vi "PointGrey Grasshopper_Settings.vi"(0 "Camera References":T4[](array[typedef]), 1 "Offset and gain":dbl[][](array[numeric]), 5 "Camera to address":i32 min=0 max=1 step=1, 7 "Camera orientation":T3(array[ring])=[enum."No rotation, No flip", enum."No rotation, No flip", enum."No rotation, Flip LR"], 9 "Which cameras record":bool[](array[boolean]), 11 "RGB Channels in":T2(array[ring]), 12 "Image buffers":T1[](array[typedef])) -> (3 "Offset gain out":dbl[][](array[numeric]), 6 "Camera to address out":i32, 8 "Camera orientation out":T3(array[ring])=[enum."No rotation, No flip", enum."No rotation, No flip", enum."No rotation, Flip LR"], 10 "Which cameras record out":bool[](array[boolean]), 15 "RGB Channels out":T2(array[ring]))   [LabVIEW 2018]
uses:
  <vilib>/userdefined/High Color/IMAQdx.ctl
  <vilib>/vision/Image Controls.llb/IMAQ Image.ctl
  <vilib>/Utility/miscctls.llb/LVOutOfRangeActionTypeDef.ctl
  <vilib>/vision/driver/IMAQdx.llb/IMAQdx Attribute Visibility.ctl
  <vilib>/vision/driver/NI_Vision_Acquisition_Software.lvlib
  <resource>/objmgr/imaqdx.rc
panel:
  in  "Tab Control":enum32{"Settings", "RGB"}(tab)
  in  "Refresh":bool
  in  "Tree":string(tree)
  in  "CameraU32":u32
  in  "CameraI64":i64
  in  "CameraDBL":dbl
  in  "CameraString":string
  in  "CameraBool":bool
  in  "CameraEnum":u16(ring) items=["Off", "Once", "Continuous"]
  in  "CameraCommand":string
  in  "Autorange Blue":bool
  in  "Autorange Green":bool
  in  "Autorange Red":bool
  in  "OK Button":bool
  # "Camera 0 is RGB, Camera 1,2... are individual cameras"
  # "Offset"
  # "Gain"
  # "Red"
  # "Green"
  # "Blue"
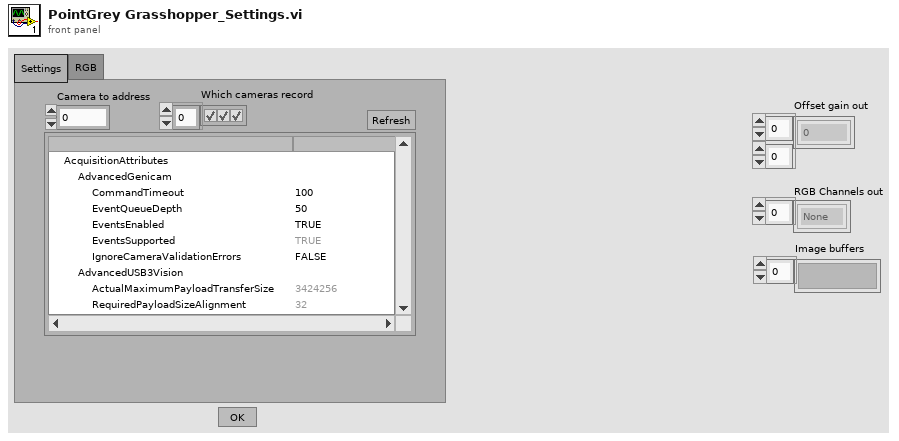
[diagram p1: front panel]
types:
  T1 = typedef "IMAQ Image.ctl" = refnum<image>
  T2 = enum16{"None", "Camera 1", "Camera 2", "Camera 3"}[]
  T3 = enum16{"No rotation, No flip", "No rotation, Flip UD", "No rotation, Flip LR", "Clockwise, No flip", "Clockwise, Flip UD", "Clockwise, Flip LR", "Anticlockwise, No flip", "Anticlockwise, Flip UD", "Anticlockwise, Flip LR"}[]
  T4 = typedef "IMAQdx.ctl" = refnum<k21>
  T5 = typedef "LVOutOfRangeActionTypeDef.ctl" = cluster{"Out of Range Action Minimum":u8, "Out of Range Action Maximum":u8, "Out of Range Action Increment":u8}
  T6 = typedef "NI_Vision_Acquisition_Software.lvlib/IMAQdx Attribute Visibility.ctl" = enum32{"Simple", "Intermediate", "Advanced"}
  T7 = enum8{"Enabled", "Disabled", "Disabled and Grayed Out"}
  T8 = typedef "NI_Vision_Acquisition_Software.lvlib/IMAQdx Attribute Type.ctl" = enum32{"U32", "I64", "DBL", "String", "Enum", "Bool", "Command"}
  T9 = cluster{"Attribute Type":T8, "Readable":bool, "Writable":bool, "Attribute Name":string}[]
  T10 = enum16{"None", "Camera 1", "Camera 2", "Camera 3"}
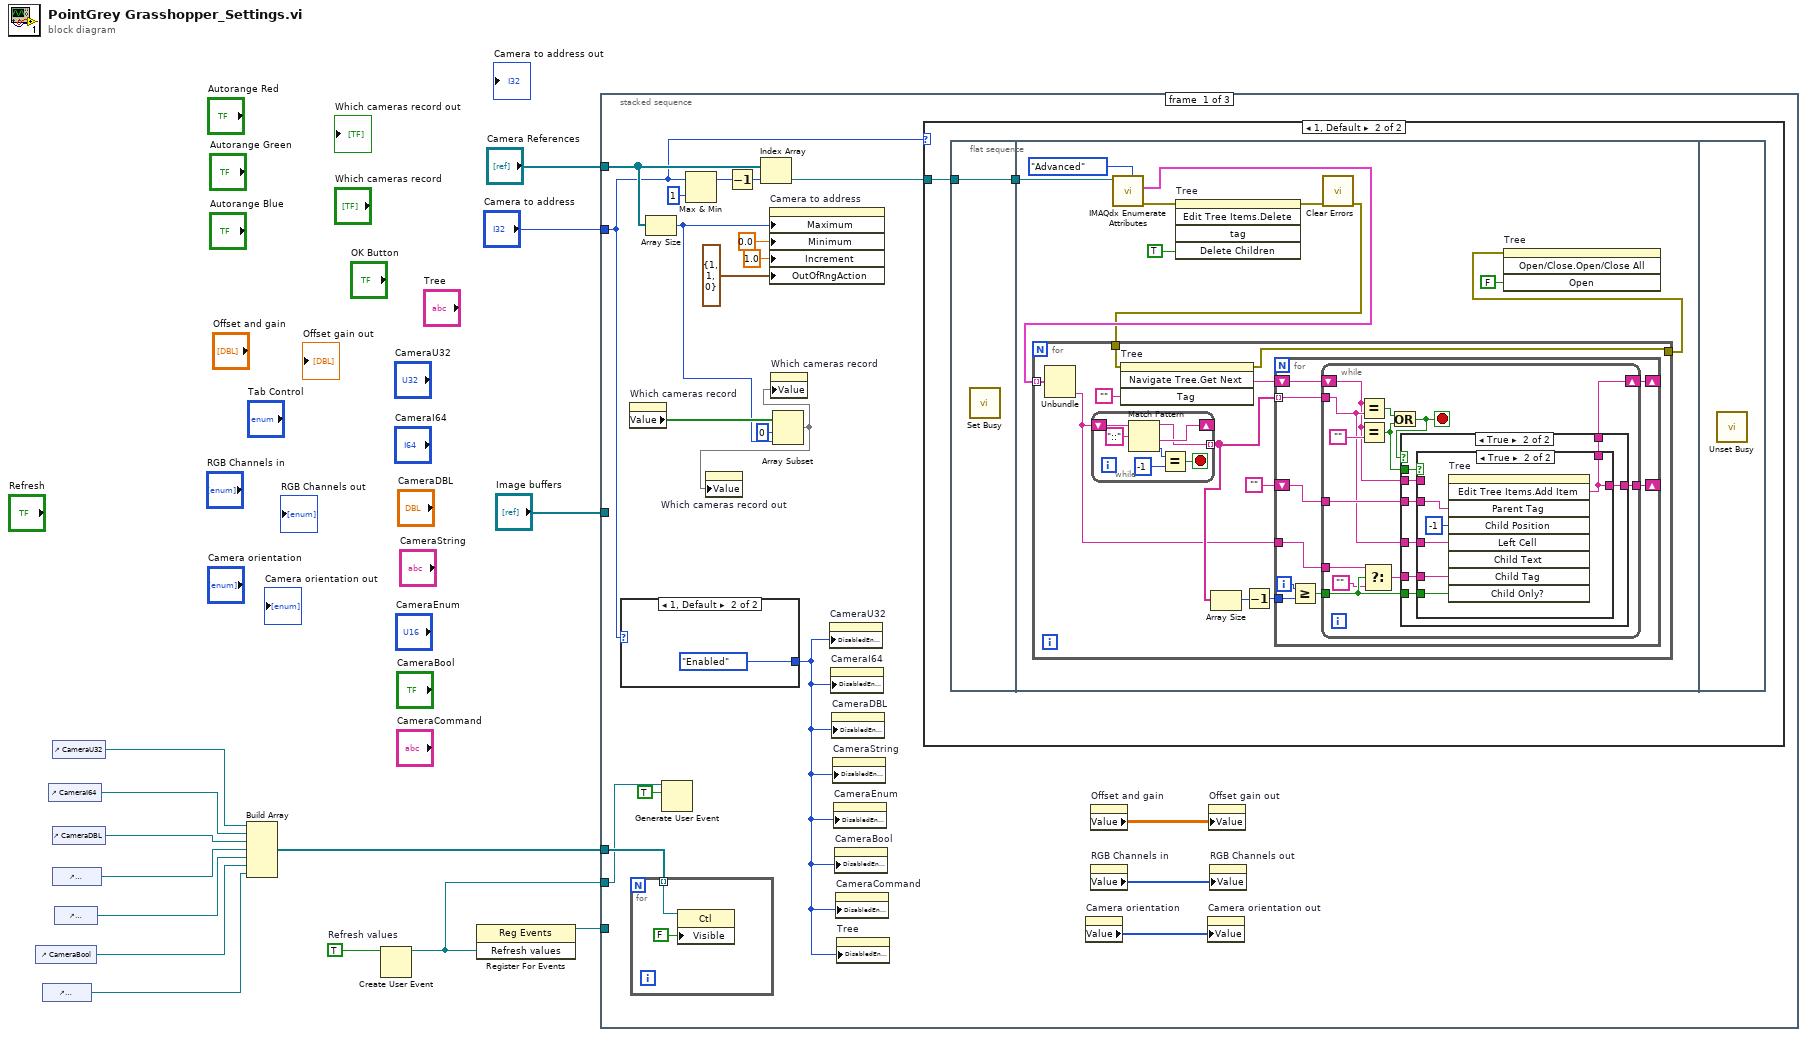
[diagram p0: block diagram]
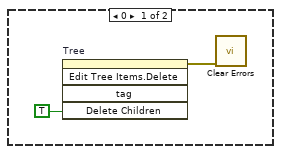
[diagram p2: hidden frame]
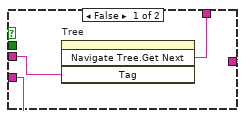
[diagram p3: hidden frame]
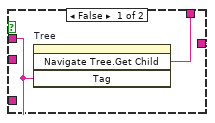
[diagram p4: hidden frame]
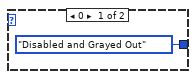
[diagram p5: hidden frame]
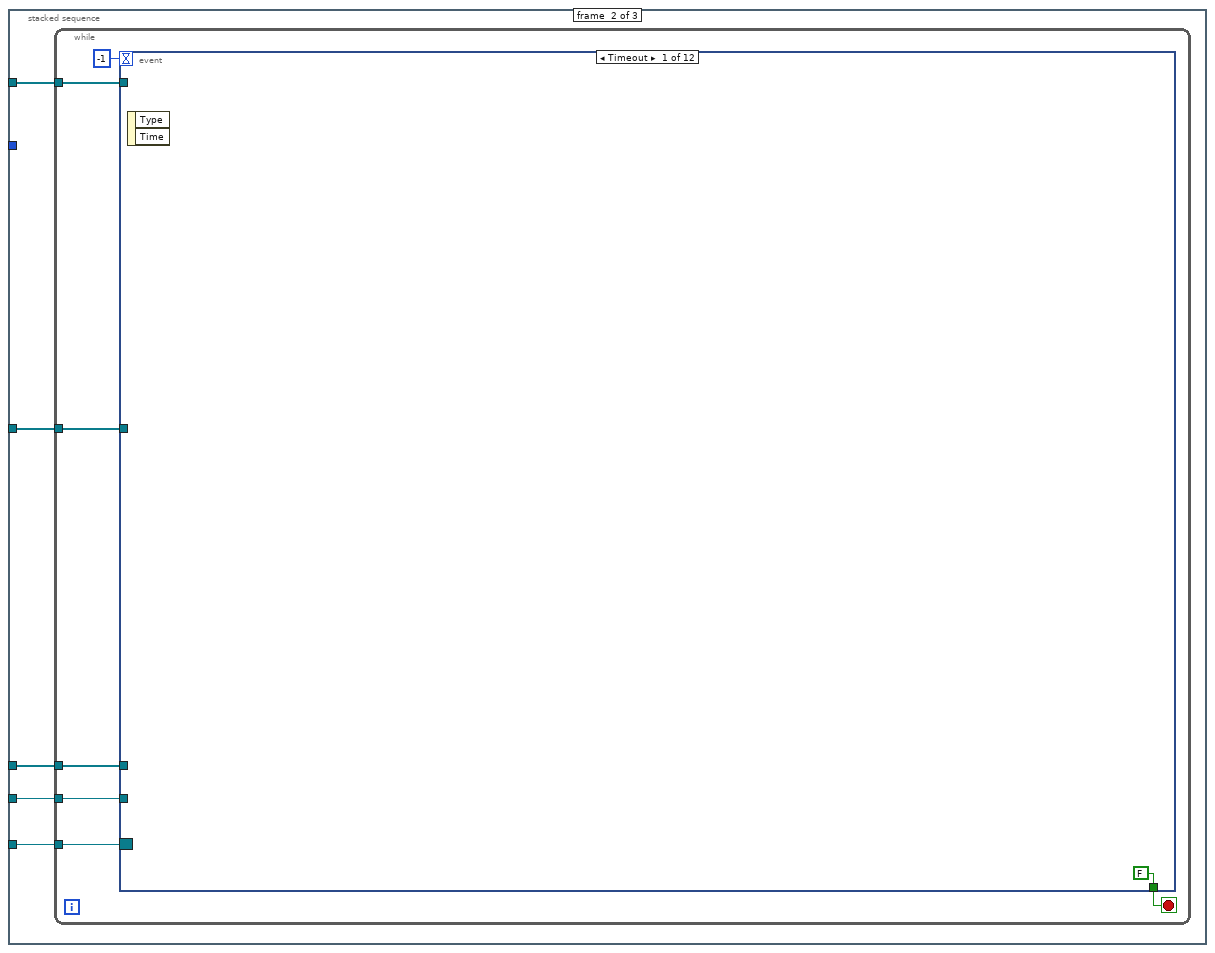
[diagram p6: hidden frame]
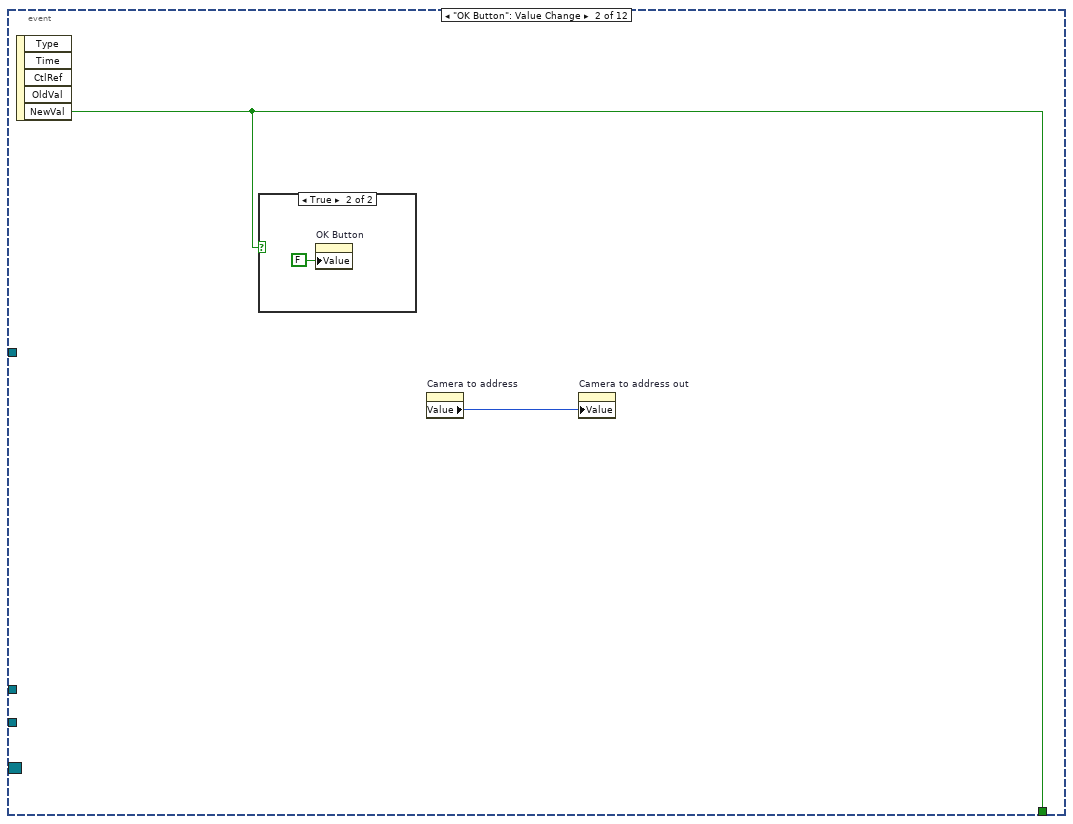
[diagram p7: hidden frame]
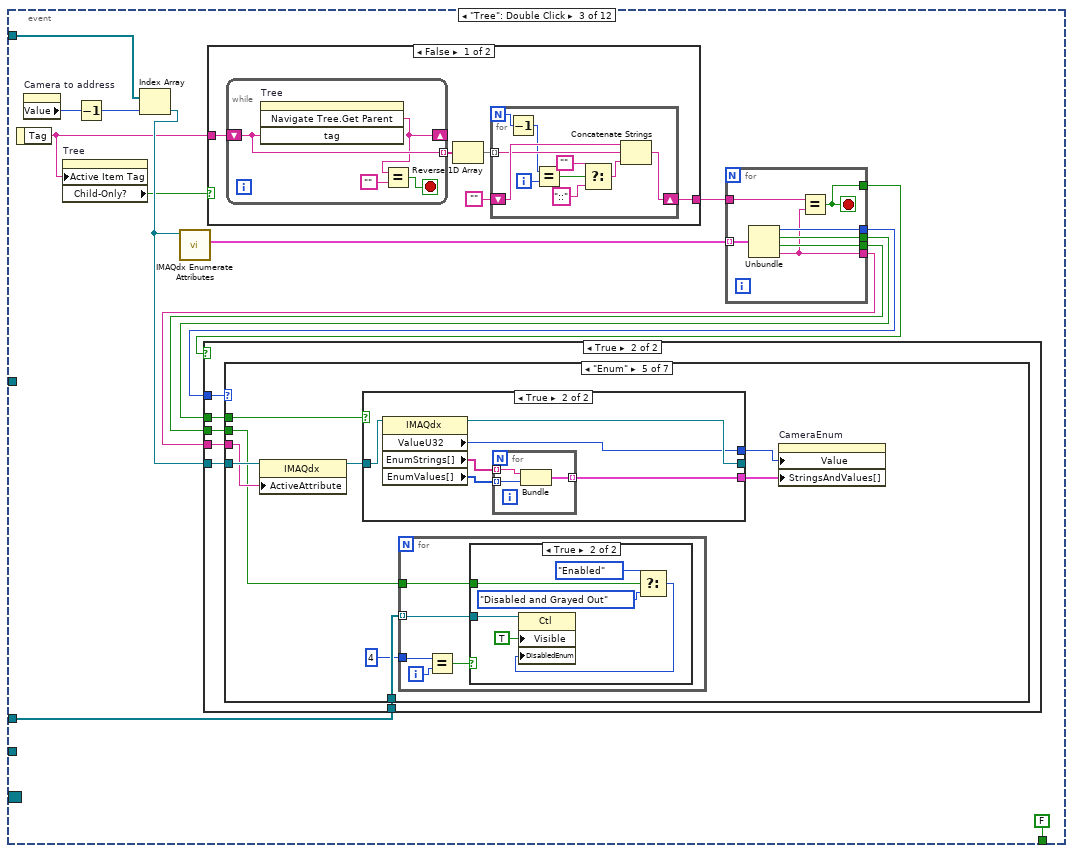
[diagram p9: hidden frame]
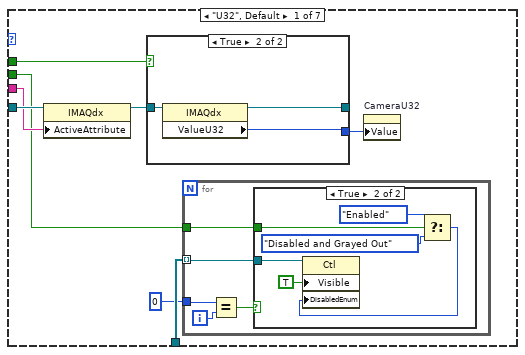
[diagram p12: hidden frame]
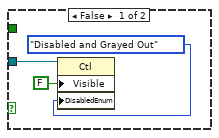
[diagram p13: hidden frame]
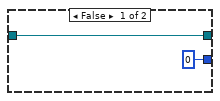
[diagram p14: hidden frame]
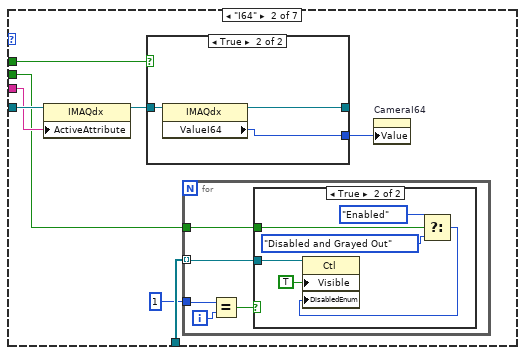
[diagram p15: hidden frame]
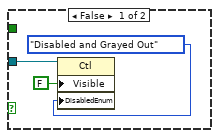
[diagram p16: hidden frame]
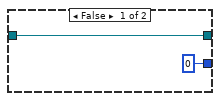
[diagram p17: hidden frame]
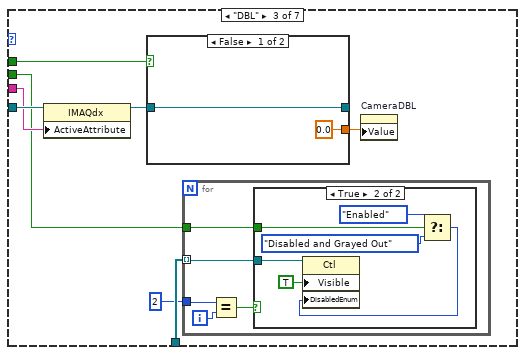
[diagram p18: hidden frame]
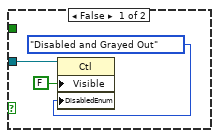
[diagram p19: hidden frame]
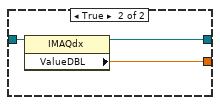
[diagram p20: hidden frame]
diagram:
  w2 = TRUE  # Refresh values
  n1 = control-ref of="CameraBool"() -> (w7:refnum<vi>)
  n2 = control-ref of="CameraCommand"() -> (w6:refnum<vi>)
  n3 = control-ref of="CameraI64"() -> (w11:refnum<vi>)
  n4 = control-ref of="CameraU32"() -> (w12:refnum<vi>)
  n5 = control-ref of="CameraDBL"() -> (w10:refnum<vi>)
  n6 = control-ref of="CameraString"() -> (w9:refnum<vi>)
  n7 = control-ref of="CameraEnum"() -> (w8:refnum<vi>)
  n8 = Build Array(w12, w11, w10, w9, w8, w7, w6) -> (w5:refnum<vi>[])
  n9 = Create User Event(user event datatype=w2) -> (user event=w1:refnum<user-event>)  [unwired: 1 in, 1 out]
  n10 = register-events(w1) -> (reference out=w3:refnum<event-registration>)  [unwired: 2 in, 1 out]
  n11 = stacked-sequence {
    tunnel: "Camera References" -> [w32 w115 _]
    tunnel: "Camera to address" -> [w15 _ _]
    tunnel: w5 -> [w33 w114 _]
    tunnel: "Image buffers" -> [_ w113 _]
    tunnel: w3 -> [_ w112 _]
    tunnel: w1 -> [w21 w111 w650]
    frame #0 {
      n12 = case shown="1, Default" w15 {
        tunnel: [T7."Disabled and Grayed Out" ("Disabled") T7."Enabled" ("Disabled")] -> w26
        frame 0 {
        }
        frame 1, Default {
        }
      }
      n13 = property on="Which cameras record" class="Arr (strict)"() -> ("Value"=w27:bool[])  [unwired: 2 in, 2 out]
      n14 = for {
        tunnel: w33 -> [w110] mode=indexing
        n15 = property class="Ctl"(reference=w110, "Visible"=FALSE) -> ()  [unwired: 1 in, 2 out]
      }
      n16 = Array Size(array=w32) -> (size(s)=w22:i32)
      n17 = Generate User Event(user event=w21, event data cluster=TRUE ("event data")) -> ()  [unwired: 2 in, 2 out]
      n18 = Max & Min(x=w15, y=1) -> (max(x,y)=w17:i32)  [unwired: 1 out]
      n19 = Decrement(x=w17) -> (x-1=w19:i32)
      n20 = Index Array(array=w32, index=w19) -> (element=w34:T4)
      n21 = property on="Camera to address" class="DigNum (strict)"("Maximum"=w22, "Minimum"=0.0 ("Data Entry Limits:Minimum"), "Increment"=1.0 ("Data Entry Limits:Increment"), "OutOfRngAction"=T5 {"Out of Range Action Minimum"=1, "Out of Range Action Maximum"=1, "Out of Range Action Increment"=0} ("Response to Value Outside Limits")) -> ()  [unwired: 2 in, 2 out]
      n22 = Array Subset(array=w27, index=0, length=w22) -> (w18:bool[])
      n23 = property on="Which cameras record out" class="Arr (strict)"("Value"=w18) -> ()  [unwired: 2 in, 2 out]
      n24 = property on="Which cameras record" class="Arr (strict)"("Value"=w18) -> ()  [unwired: 2 in, 2 out]
      n25 = property on="CameraU32" class="DigNum (strict)"("DisabledEnum"=w26) -> ()  [unwired: 2 in, 2 out]
      n26 = property on="CameraI64" class="DigNum (strict)"("DisabledEnum"=w26) -> ()  [unwired: 2 in, 2 out]
      n27 = property on="CameraDBL" class="DigNum (strict)"("DisabledEnum"=w26) -> ()  [unwired: 2 in, 2 out]
      n28 = property on="CameraString" class="Str"("DisabledEnum"=w26) -> ()  [unwired: 2 in, 2 out]
      n29 = property on="CameraEnum" class="Ring (strict)"("DisabledEnum"=w26) -> ()  [unwired: 2 in, 2 out]
      n30 = property on="CameraBool" class="Bool (strict)"("DisabledEnum"=w26) -> ()  [unwired: 2 in, 2 out]
      n31 = property on="CameraCommand" class="Str"("DisabledEnum"=w26) -> ()  [unwired: 2 in, 2 out]
      n32 = property on="Tree" class="Tree (strict)"("DisabledEnum"=w26) -> ()  [unwired: 2 in, 2 out]
      n33 = case shown="1, Default" w15 {
        tunnel: w34 -> [_ w38]
        frame 0 {
          n34 = invoke on="Tree" class="Tree (strict)" method="Edit Tree Items.Delete"("Delete Children"=TRUE ("Delete Children?")) -> (error out=w35:errorcluster)  [unwired: 4 in, 4 out]
          n35 = call <vilib>:"Clear Errors.vi"("error in (no error)"=w35) -> ()  [unwired: 5 in, 2 out]
        }
        frame 1, Default {
          n36 = flat-sequence {
            tunnel: w38 -> [w39]
            tunnel: [w39] -> w37
            tunnel: w37 -> [w40]
            frame #0 {
              n37 = call <vilib>:"Set Busy.vi"() -> ()  [unwired: 10 in, 2 out]
            }
            frame #1 {
              n38 = call <vilib>:"IMAQdx Enumerate Attributes.vi"("Visibility"=IMAQdx_Attribute_Visibility."Advanced", "Session In"=w40) -> ("error out"=w44:errorcluster, "Attribute Information Array"=w48:T9)  [unwired: 7 in, 1 out]
              n39 = invoke on="Tree" class="Tree (strict)" method="Edit Tree Items.Delete"(error in=w44, "Delete Children"=TRUE ("Delete Children?")) -> (error out=w43:errorcluster)  [unwired: 3 in, 4 out]
              n40 = call <vilib>:"Clear Errors.vi"("error in (no error)"=w43) -> ("error out"=w45:errorcluster)  [unwired: 5 in, 1 out]
              n41 = for {
                tunnel: w48 -> [w58] mode=indexing
                tunnel: w45 -> [w51]
                tunnel: [w50] -> w47
                n42 = Unbundle(w58) -> ("Attribute Name"=w49:string)  [unwired: 3 out]
                n43 = while {
                  shift-right: [w104] -> _
                  shift-left: w49 -> [w106]
                  tunnel: [w100] -> w55 mode=indexing
                  stop <- w101 stop-if-true
                  n44 = Match Pattern(string=w106, regular expression="::") -> (before substring=w100:string, after substring=w104:string, offset past match=w103:i32)  [unwired: 1 in, 1 out]
                  n45 = Equal?(x=w103, y=-1) -> (x = y?=w101:bool)
                }
                n46 = invoke on="Tree" class="Tree (strict)" method="Navigate Tree.Get Next"(error in=w51, "Tag"="") -> (error out=w50:errorcluster, "Navigate Tree:Get Next Item"=w53:string)  [unwired: 2 in, 2 out]
                n47 = Array Size(array=w55) -> (size(s)=w56:i32)
                n48 = Decrement(x=w56) -> (x-1=w52:i32)
                n49 = for {
                  tunnel: w55 -> [w67] mode=indexing
                  shift-right: [w66] -> _
                  shift-left: "" -> [w65]
                  tunnel: w52 -> [w63]
                  shift-right: [w60] -> _
                  shift-left: w53 -> [w61]
                  tunnel: w49 -> [w59]
                  i -> [w62]
                  n50 = Greater Or Equal?(x=w62, y=w63) -> (x >= y?=w64:bool)
                  n51 = while {
                    shift-right: [w72] -> w60
                    shift-left: w61 -> [w73]
                    tunnel: w67 -> [w74]
                    tunnel: [w76] -> w66
                    tunnel: w65 -> [w75]
                    tunnel: w64 -> [w71]
                    tunnel: w59 -> [w69]
                    stop <- w78 stop-if-true
                    n52 = Equal?(x=w73, y=w74) -> (x = y?=w79:bool)
                    n53 = Equal?(x=w73, y="") -> (x = y?=w77:bool)
                    n54 = Select(t=w69, s=w71, f="") -> (s? t:f=w70:string)
                    n55 = Or(x=w79, y=w77) -> (x .or. y?=w78:bool)
                    n56 = case shown="True" w78 {
                      tunnel: w73 -> [w82 w90]
                      tunnel: w77 -> [_ w91]
                      tunnel: [w83 w89] -> w76
                      tunnel: w75 -> [w83 w88]
                      tunnel: w71 -> [_ w87]
                      tunnel: w74 -> [_ w86]
                      tunnel: [w81 w85] -> w72
                      tunnel: w70 -> [_ w84]
                      frame False {
                        n57 = invoke on="Tree" class="Tree (strict)" method="Navigate Tree.Get Next"("Tag"=w82) -> ("Navigate Tree:Get Next Item"=w81:string)  [unwired: 3 in, 3 out]
                      }
                      frame True {
                        n58 = case shown="True" w91 {
                          tunnel: w90 -> [w92 _]
                          tunnel: [w92 w95] -> w89
                          tunnel: w88 -> [_ w96]
                          tunnel: w87 -> [_ w98]
                          tunnel: w86 -> [_ w97]
                          tunnel: [w93 w95] -> w85
                          tunnel: w84 -> [_ w94]
                          frame False {
                            n59 = invoke on="Tree" class="Tree (strict)" method="Navigate Tree.Get Child"("Tag"=w92) -> ("Navigate Tree:Get Child"=w93:string)  [unwired: 3 in, 3 out]
                          }
                          frame True {
                            n60 = invoke on="Tree" class="Tree (strict)" method="Edit Tree Items.Add Item"("Parent Tag"=w96, "Child Position"=-1, "Left Cell"=w97, "Child Tag"=w94, "Child Only?"=w98) -> ("Edit Tree Items:Add Item"=w95:string)  [unwired: 4 in, 8 out]
                          }
                        }
                      }
                    }
                  }
                }
              }
              n61 = invoke on="Tree" class="Tree (strict)" method="Open/Close.Open/Close All"(error in=w47, "Open"=FALSE ("Open?")) -> ()  [unwired: 2 in, 4 out]
            }
            frame #2 {
              n62 = call <vilib>:"Unset Busy.vi"() -> ()  [unwired: 11 in, 1 out]
            }
          }
        }
      }
      n63 = property on="Camera orientation" class="Arr (strict)"() -> ("Value"=w16:T3)  [unwired: 2 in, 2 out]
      n64 = property on="Offset and gain" class="Arr (strict)"() -> ("Value"=w24:dbl[][])  [unwired: 2 in, 2 out]
      n65 = property on="RGB Channels in" class="Arr (strict)"() -> ("Value"=w23:T2)  [unwired: 2 in, 2 out]
      n66 = property on="Camera orientation out" class="Arr (strict)"("Value"=w16) -> ()  [unwired: 2 in, 2 out]
      n67 = property on="Offset gain out" class="Arr (strict)"("Value"=w24) -> ()  [unwired: 2 in, 2 out]
      n68 = property on="RGB Channels out" class="Arr (strict)"("Value"=w23) -> ()  [unwired: 2 in, 2 out]
    }
    frame #1 {
      n69 = while {
        tunnel: w115 -> [w120]
        tunnel: w114 -> [w119]
        tunnel: w113 -> [w118]
        tunnel: w112 -> [w117]
        tunnel: w111 -> [w116]
        stop <- w121 stop-if-true
        n70 = event shown="[0] Timeout" {
          selector: w117 -> [_ _ _ _ _ _ _ _ _ _ _ _]
          dyn-events: _ -> [_ _ _ _ _ _ _ _ _ _ _ _]
          timeout: -1 -> [_ _ _ _ _ _ _ _ _ _ _ _]
          tunnel: [FALSE ("NewVal") w125 FALSE ("NewVal") FALSE ("NewVal") FALSE ("NewVal") FALSE ("NewVal") FALSE ("NewVal") FALSE ("NewVal") FALSE ("NewVal") FALSE ("NewVal") FALSE ("NewVal") FALSE ("NewVal")] -> w121
          tunnel: w120 -> [_ _ w134 w373 w458 w464 _ _ _ _ w598 _]
          tunnel: w119 -> [_ _ w131 _ _ _ _ _ _ _ w600 _]
          tunnel: w118 -> [_ _ _ _ _ _ _ _ _ w553 _ _]
          tunnel: w116 -> [_ _ _ _ _ w460 _ _ _ _ w596 w645]
          event Timeout {
            n71 = event-data() -> ()  [unwired: 1 in, 2 out]
          }
          event "OK Button": Value Change {
            n72 = event-data() -> ("NewVal"=w125:bool)  [unwired: 1 in, 4 out]
            n73 = case shown="True" w125 {
              frame False {
              }
              frame True {
                n74 = property on="OK Button" class="Bool (strict)"("Value"=FALSE ("OK Button")) -> ()  [unwired: 2 in, 2 out]
              }
            }
            n75 = property on="Camera to address" class="DigNum (strict)"() -> ("Value"=w124:i32)  [unwired: 2 in, 2 out]
            n76 = property on="Camera to address out" class="DigNum (strict)"("Value"=w124) -> ()  [unwired: 2 in, 2 out]
          }
          event "Tree": Double Click {
            n77 = event-data() -> ("Tag"=w128:string)  [unwired: 1 in]
            n78 = property on="Camera to address" class="DigNum (strict)"() -> ("Value"=w133:i32)  [unwired: 2 in, 2 out]
            n79 = property on="Tree" class="Tree (strict)"("Active Item Tag"=w128) -> ("Child-Only?"=w127:bool)  [unwired: 2 in, 2 out]
            n80 = Decrement(x=w133) -> (x-1=w129:i32)
            n81 = Index Array(array=w134, index=w129) -> (element=w132:T4)
            n82 = call <vilib>:"IMAQdx Enumerate Attributes.vi"("Session In"=w132) -> ("Attribute Information Array"=w135:T9)  [unwired: 8 in, 2 out]
            n83 = case shown="False" w127 {
              tunnel: [w143 w161] -> w141
              tunnel: w128 -> [w142 w161]
              frame False {
                n84 = while {
                  shift-right: [w149] -> _
                  shift-left: w142 -> [w150]
                  tunnel: [w150] -> w146 mode=indexing
                  stop <- w147 stop-if-true
                  n85 = invoke on="Tree" class="Tree (strict)" method="Navigate Tree.Get Parent"("tag"=w150) -> ("Navigate Tree:Get Parent"=w149:string)  [unwired: 3 in, 3 out]
                  n86 = Equal?(x=w149, y="") -> (x = y?=w147:bool)
                }
                n87 = Reverse 1D Array(array=w146) -> (reversed array=w144:string[])
                n88 = for {
                  N -> [w157]
                  tunnel: w144 -> [w159] mode=indexing
                  shift-right: [w151] -> w143
                  shift-left: "" -> [w160]
                  i -> [w154]
                  n89 = Decrement(x=w157) -> (x-1=w155:i32)
                  n90 = Equal?(x=w155, y=w154) -> (x = y?=w156:bool)
                  n91 = Select(t="", s=w156, f="::" ("t")) -> (s? t:f=w158:string)
                  n92 = Concatenate Strings(w160, w159, w158) -> (w151:string)
                }
              }
              frame True {
              }
            }
            n93 = for {
              tunnel: w135 -> [w371] mode=indexing
              tunnel: w141 -> [w370]
              tunnel: [w369] -> w137
              tunnel: [w368] -> w138
              tunnel: [w367] -> w139
              tunnel: [w366] -> w140
              tunnel: [w365] -> w136
              stop <- w366 stop-if-true
              n94 = Unbundle(w371) -> ("Attribute Type"=w367:T8, "Readable"=w368:bool, "Writable"=w369:bool, "Attribute Name"=w365:string)
              n95 = Equal?(x=w370, y=w365) -> (x = y?=w366:bool)
            }
            n96 = case shown="True" w140 {
              tunnel: w139 -> [_ w167]
              tunnel: w138 -> [_ w166]
              tunnel: w137 -> [_ w165]
              tunnel: w136 -> [_ w164]
              tunnel: w132 -> [_ w163]
              tunnel: w131 -> [_ w162]
              frame False {
              }
              frame True {
                n97 = case shown="\"Enum\"" w167 {
                  tunnel: w166 -> [w169 w196 w223 w250 w277 w312 w339]
                  tunnel: w165 -> [w168 w195 w222 w249 w276 w311 w338]
                  tunnel: w164 -> [w174 w201 w228 w255 w283 w317 w344]
                  tunnel: w163 -> [w175 w202 w229 w256 w284 w318 w345]
                  tunnel: w162 -> [w172 w199 w226 w253 w281 w315 w342]
                  frame "U32", Default {
                    n98 = property class="IMAQdx"(reference=w175, "ActiveAttribute"=w174) -> (reference out=w173:T4)  [unwired: 1 in, 1 out]
                    n99 = case shown="True" w169 {
                      tunnel: w173 -> [w191 w194]
                      tunnel: [w191 w193] -> _
                      tunnel: [u32 0 ("ValueU32") w192] -> w170
                      frame False {
                      }
                      frame True {
                        n100 = property class="IMAQdx"(reference=w194) -> (reference out=w193:T4, "ValueU32"=w192:u32)  [unwired: 1 in, 1 out]
                      }
                    }
                    n101 = for {
                      tunnel: w172 -> [w180] mode=indexing
                      tunnel: 0 -> [w177]
                      tunnel: w168 -> [w176]
                      i -> [w179]
                      n102 = Equal?(x=w177, y=w179) -> (x = y?=w178:bool)
                      n103 = case shown="True" w178 {
                        tunnel: w180 -> [w183 w189]
                        tunnel: w176 -> [_ w187]
                        frame False {
                          n104 = property class="Ctl"(reference=w183, "Visible"=FALSE, "DisabledEnum"=T7."Disabled and Grayed Out" ("Disabled")) -> ()  [unwired: 1 in, 2 out]
                        }
                        frame True {
                          n105 = Select(t=T7."Enabled" ("Disabled"), s=w187, f=T7."Disabled and Grayed Out" ("Disabled")) -> (s? t:f=w184:T7)
                          n106 = property class="Ctl"(reference=w189, "Visible"=TRUE, "DisabledEnum"=w184) -> ()  [unwired: 1 in, 2 out]
                        }
                      }
                    }
                    n107 = property on="CameraU32" class="DigNum (strict)"("Value"=w170) -> ()  [unwired: 2 in, 2 out]
                  }
                  frame "I64" {
                    n108 = property class="IMAQdx"(reference=w202, "ActiveAttribute"=w201) -> (reference out=w200:T4)  [unwired: 1 in, 1 out]
                    n109 = case shown="True" w196 {
                      tunnel: w200 -> [w218 w221]
                      tunnel: [w218 w220] -> _
                      tunnel: [i64 0 ("ValueI64") w219] -> w197
                      frame False {
                      }
                      frame True {
                        n110 = property class="IMAQdx"(reference=w221) -> (reference out=w220:T4, "ValueI64"=w219:i64)  [unwired: 1 in, 1 out]
                      }
                    }
                    n111 = for {
                      tunnel: w199 -> [w207] mode=indexing
                      tunnel: 1 -> [w204]
                      tunnel: w195 -> [w203]
                      i -> [w206]
                      n112 = Equal?(x=w204, y=w206) -> (x = y?=w205:bool)
                      n113 = case shown="True" w205 {
                        tunnel: w207 -> [w210 w216]
                        tunnel: w203 -> [_ w214]
                        frame False {
                          n114 = property class="Ctl"(reference=w210, "Visible"=FALSE, "DisabledEnum"=T7."Disabled and Grayed Out" ("Disabled")) -> ()  [unwired: 1 in, 2 out]
                        }
                        frame True {
                          n115 = Select(t=T7."Enabled" ("Disabled"), s=w214, f=T7."Disabled and Grayed Out" ("Disabled")) -> (s? t:f=w211:T7)
                          n116 = property class="Ctl"(reference=w216, "Visible"=TRUE, "DisabledEnum"=w211) -> ()  [unwired: 1 in, 2 out]
                        }
                      }
                    }
                    n117 = property on="CameraI64" class="DigNum (strict)"("Value"=w197) -> ()  [unwired: 2 in, 2 out]
                  }
                  frame "DBL" {
                    n118 = property class="IMAQdx"(reference=w229, "ActiveAttribute"=w228) -> (reference out=w227:T4)  [unwired: 1 in, 1 out]
                    n119 = case shown="False" w223 {
                      tunnel: w227 -> [w245 w248]
                      tunnel: [w245 w247] -> _
                      tunnel: [0.0 ("ValueDBL") w246] -> w224
                      frame False {
                      }
                      frame True {
                        n120 = property class="IMAQdx"(reference=w248) -> (reference out=w247:T4, "ValueDBL"=w246:dbl)  [unwired: 1 in, 1 out]
                      }
                    }
                    n121 = for {
                      tunnel: w226 -> [w234] mode=indexing
                      tunnel: 2 -> [w231]
                      tunnel: w222 -> [w230]
                      i -> [w233]
                      n122 = Equal?(x=w231, y=w233) -> (x = y?=w232:bool)
                      n123 = case shown="True" w232 {
                        tunnel: w234 -> [w237 w243]
                        tunnel: w230 -> [_ w241]
                        frame False {
                          n124 = property class="Ctl"(reference=w237, "Visible"=FALSE, "DisabledEnum"=T7."Disabled and Grayed Out" ("Disabled")) -> ()  [unwired: 1 in, 2 out]
                        }
                        frame True {
                          n125 = Select(t=T7."Enabled" ("Disabled"), s=w241, f=T7."Disabled and Grayed Out" ("Disabled")) -> (s? t:f=w238:T7)
                          n126 = property class="Ctl"(reference=w243, "Visible"=TRUE, "DisabledEnum"=w238) -> ()  [unwired: 1 in, 2 out]
                        }
                      }
                    }
                    n127 = property on="CameraDBL" class="DigNum (strict)"("Value"=w224) -> ()  [unwired: 2 in, 2 out]
                  }
                  frame "String" {
                    n128 = property class="IMAQdx"(reference=w256, "ActiveAttribute"=w255) -> (reference out=w254:T4)  [unwired: 1 in, 1 out]
                    n129 = case shown="False" w250 {
                      tunnel: w254 -> [w272 w275]
                      tunnel: [w272 w274] -> _
                      tunnel: ["" ("ValueString") w273] -> w251
                      frame False {
                      }
                      frame True {
                        n130 = property class="IMAQdx"(reference=w275) -> (reference out=w274:T4, "ValueString"=w273:string)  [unwired: 1 in, 1 out]
                      }
                    }
                    n131 = for {
                      tunnel: w253 -> [w261] mode=indexing
                      tunnel: 3 -> [w258]
                      tunnel: w249 -> [w257]
                      i -> [w260]
                      n132 = Equal?(x=w258, y=w260) -> (x = y?=w259:bool)
                      n133 = case shown="True" w259 {
                        tunnel: w261 -> [w264 w270]
                        tunnel: w257 -> [_ w268]
                        frame False {
                          n134 = property class="Ctl"(reference=w264, "Visible"=FALSE, "DisabledEnum"=T7."Disabled and Grayed Out" ("Disabled")) -> ()  [unwired: 1 in, 2 out]
                        }
                        frame True {
                          n135 = Select(t=T7."Enabled" ("Disabled"), s=w268, f=T7."Disabled and Grayed Out" ("Disabled")) -> (s? t:f=w265:T7)
                          n136 = property class="Ctl"(reference=w270, "Visible"=TRUE, "DisabledEnum"=w265) -> ()  [unwired: 1 in, 2 out]
                        }
                      }
                    }
                    n137 = property on="CameraString" class="Str"("Value"=w251) -> ()  [unwired: 2 in, 2 out]
                  }
                  frame "Enum" {
                    n138 = property class="IMAQdx"(reference=w284, "ActiveAttribute"=w283) -> (reference out=w282:T4)  [unwired: 1 in, 1 out]
                    n139 = case shown="True" w277 {
                      tunnel: w282 -> [w301 w307]
                      tunnel: [w301 w306] -> _
                      tunnel: [u32 0 ("ValueU32") w303] -> w279
                      tunnel: [cluster{string, u32}[] [] w302] -> w278
                      frame False {
                      }
                      frame True {
                        n140 = property class="IMAQdx"(reference=w307) -> (reference out=w306:T4, "ValueU32"=w303:u32, "EnumStrings[]"=w305:string[], "EnumValues[]"=w304:u32[])  [unwired: 1 in, 1 out]
                        n141 = for {
                          tunnel: w305 -> [w309] mode=indexing
                          tunnel: w304 -> [w310] mode=indexing
                          tunnel: [w308] -> w302 mode=indexing
                          n142 = Bundle(w309, w310) -> (w308:cluster{string, u32})  [unwired: 1 in]
                        }
                      }
                    }
                    n143 = for {
                      tunnel: w281 -> [w289] mode=indexing
                      tunnel: 4 -> [w286]
                      tunnel: w276 -> [w285]
                      i -> [w288]
                      n144 = Equal?(x=w286, y=w288) -> (x = y?=w287:bool)
                      n145 = case shown="True" w287 {
                        tunnel: w289 -> [w292 w298]
                        tunnel: w285 -> [_ w296]
                        frame False {
                          n146 = property class="Ctl"(reference=w292, "Visible"=FALSE, "DisabledEnum"=T7."Disabled and Grayed Out" ("Disabled")) -> ()  [unwired: 1 in, 2 out]
                        }
                        frame True {
                          n147 = Select(t=T7."Enabled" ("Disabled"), s=w296, f=T7."Disabled and Grayed Out" ("Disabled")) -> (s? t:f=w293:T7)
                          n148 = property class="Ctl"(reference=w298, "Visible"=TRUE, "DisabledEnum"=w293) -> ()  [unwired: 1 in, 2 out]
                        }
                      }
                    }
                    n149 = property on="CameraEnum" class="Ring (strict)"("Value"=w279, "StringsAndValues[]"=w278) -> ()  [unwired: 2 in, 2 out]
                  }
                  frame "Bool" {
                    n150 = property class="IMAQdx"(reference=w318, "ActiveAttribute"=w317) -> (reference out=w316:T4)  [unwired: 1 in, 1 out]
                    n151 = case shown="False" w312 {
                      tunnel: w316 -> [w334 w337]
                      tunnel: [w334 w336] -> _
                      tunnel: [FALSE ("ValueBool") w335] -> w313
                      frame False {
                      }
                      frame True {
                        n152 = property class="IMAQdx"(reference=w337) -> (reference out=w336:T4, "ValueBool"=w335:bool)  [unwired: 1 in, 1 out]
                      }
                    }
                    n153 = for {
                      tunnel: w315 -> [w323] mode=indexing
                      tunnel: 5 -> [w320]
                      tunnel: w311 -> [w319]
                      i -> [w322]
                      n154 = Equal?(x=w320, y=w322) -> (x = y?=w321:bool)
                      n155 = case shown="True" w321 {
                        tunnel: w323 -> [w326 w332]
                        tunnel: w319 -> [_ w330]
                        frame False {
                          n156 = property class="Ctl"(reference=w326, "Visible"=FALSE, "DisabledEnum"=T7."Disabled and Grayed Out" ("Disabled")) -> ()  [unwired: 1 in, 2 out]
                        }
                        frame True {
                          n157 = Select(t=T7."Enabled" ("Disabled"), s=w330, f=T7."Disabled and Grayed Out" ("Disabled")) -> (s? t:f=w327:T7)
                          n158 = property class="Ctl"(reference=w332, "Visible"=TRUE, "DisabledEnum"=w327) -> ()  [unwired: 1 in, 2 out]
                        }
                      }
                    }
                    n159 = property on="CameraBool" class="Bool (strict)"("Value"=w313) -> ()  [unwired: 2 in, 2 out]
                  }
                  frame "Command" {
                    n160 = property class="IMAQdx"(reference=w345, "ActiveAttribute"=w344) -> (reference out=w343:T4)  [unwired: 1 in, 1 out]
                    n161 = case shown="True" w339 {
                      tunnel: w343 -> [w361 w364]
                      tunnel: [w361 w363] -> _
                      tunnel: ["" ("ValueString") w362] -> w340
                      frame False {
                      }
                      frame True {
                        n162 = property class="IMAQdx"(reference=w364) -> (reference out=w363:T4, "ValueString"=w362:string)  [unwired: 1 in, 1 out]
                      }
                    }
                    n163 = for {
                      tunnel: w342 -> [w350] mode=indexing
                      tunnel: 6 -> [w347]
                      tunnel: w338 -> [w346]
                      i -> [w349]
                      n164 = Equal?(x=w347, y=w349) -> (x = y?=w348:bool)
                      n165 = case shown="True" w348 {
                        tunnel: w350 -> [w353 w359]
                        tunnel: w346 -> [_ w357]
                        frame False {
                          n166 = property class="Ctl"(reference=w353, "Visible"=FALSE, "DisabledEnum"=T7."Disabled and Grayed Out" ("Disabled")) -> ()  [unwired: 1 in, 2 out]
                        }
                        frame True {
                          n167 = Select(t=T7."Enabled" ("Disabled"), s=w357, f=T7."Disabled and Grayed Out" ("Disabled")) -> (s? t:f=w354:T7)
                          n168 = property class="Ctl"(reference=w359, "Visible"=TRUE, "DisabledEnum"=w354) -> ()  [unwired: 1 in, 2 out]
                        }
                      }
                    }
                    n169 = property on="CameraCommand" class="Str"("Value"=w340) -> ()  [unwired: 2 in, 2 out]
                  }
                }
              }
            }
          }
          event User Event {
            n170 = event-data() -> ()  [unwired: 1 in, 5 out]
            n171 = property on="Camera to address" class="DigNum (strict)"() -> ("Value"=w372:i32)  [unwired: 2 in, 2 out]
            n172 = case shown="0" w372 {
              selector: w372 -> [_ w375]
              tunnel: w373 -> [_ w377]
              frame 0 {
              }
              frame 1, Default {
                n173 = Decrement(x=w375) -> (x-1=w378:i32)
                n174 = Index Array(array=w377, index=w378) -> (element=w376:T4)
                n175 = flat-sequence {
                  tunnel: w376 -> [w385]
                  tunnel: [w384] -> w382
                  tunnel: [w383] -> w381
                  tunnel: w382 -> [w386]
                  tunnel: [w387] -> w380
                  tunnel: w381 -> [w387]
                  tunnel: [w386] -> w379
                  tunnel: w380 -> [w452]
                  tunnel: w379 -> [w453]
                  frame #0 {
                    n176 = property class="IMAQdx"(reference=w385) -> (reference out=w384:T4, "ActiveAttribute"=w383:string)  [unwired: 1 in, 1 out]
                    n177 = call <vilib>:"Set Busy.vi"() -> ()  [unwired: 10 in, 2 out]
                  }
                  frame #1 {
                    n178 = call <vilib>:"IMAQdx Enumerate Attributes.vi"("Session In"=w386) -> ("Attribute Information Array"=w388:T9)  [unwired: 8 in, 2 out]
                    n179 = for {
                      tunnel: w386 -> [w397]
                      tunnel: w388 -> [w401] mode=indexing
                      n180 = Unbundle(w401) -> ("Attribute Type"=w398:T8, "Readable"=w400:bool, "Writable"=w394:bool, "Attribute Name"=w395:string)
                      n181 = Or(x=w400, y=w394) -> (x .or. y?=w399:bool)
                      n182 = case shown="True" w399 {
                        tunnel: w398 -> [_ w407]
                        tunnel: w395 -> [_ w409]
                        tunnel: w397 -> [_ w408]
                        tunnel: ["" w406] -> w396
                        tunnel: [FALSE w405] -> w393
                        frame False {
                        }
                        frame True {
                          n183 = case shown="\"Enum\"" w407 {
                            tunnel: w409 -> [w414 w419 w424 w428 w436 w447 w451]
                            tunnel: w408 -> [w413 w418 w423 w427 w435 w446 w450]
                            tunnel: [w411 w416 w421 w426 w433 w444 "<COMMAND>" ("ValueString")] -> w406
                            tunnel: [FALSE FALSE FALSE FALSE FALSE FALSE TRUE] -> w405
                            frame "U32", Default {
                              n184 = property class="IMAQdx"(reference=w413, "ActiveAttribute"=w414) -> ("ValueU32"=w412:u32)  [unwired: 1 in, 2 out]
                              n185 = Number To Decimal String(number=w412) -> (decimal integer string=w411:string)  [unwired: 1 in]
                            }
                            frame "I64" {
                              n186 = property class="IMAQdx"(reference=w418, "ActiveAttribute"=w419) -> ("ValueI64"=w417:i64)  [unwired: 1 in, 2 out]
                              n187 = Number To Decimal String(number=w417) -> (decimal integer string=w416:string)  [unwired: 1 in]
                            }
                            frame "DBL" {
                              n188 = property class="IMAQdx"(reference=w423, "ActiveAttribute"=w424) -> ("ValueDBL"=w422:dbl)  [unwired: 1 in, 2 out]
                              n189 = Number To Engineering String(4:w422) -> (0:w421:string)  [unwired: 3 in]
                            }
                            frame "String" {
                              n190 = property class="IMAQdx"(reference=w427, "ActiveAttribute"=w428) -> ("ValueString"=w426:string)  [unwired: 1 in, 2 out]
                            }
                            frame "Enum" {
                              n191 = property class="IMAQdx"(reference=w435, "ActiveAttribute"=w436) -> ("ValueU32"=w431:u32, "EnumStrings[]"=w434:string[], "EnumValues[]"=w430:u32[])  [unwired: 1 in, 2 out]
                              n192 = for {
                                tunnel: w431 -> [w438]
                                tunnel: w430 -> [w439] mode=indexing
                                tunnel: [w437] -> w429
                                i -> [w437]
                                stop <- w440 stop-if-true
                                n193 = Equal?(x=w438, y=w439) -> (x = y?=w440:bool)
                              }
                              n194 = Index Array(array=w434, index=w429) -> (element=w433:string)
                            }
                            frame "Bool" {
                              n195 = property class="IMAQdx"(reference=w446, "ActiveAttribute"=w447) -> ("ValueBool"=w445:bool)  [unwired: 1 in, 2 out]
                              n196 = Select(t="TRUE", s=w445, f="FALSE") -> (s? t:f=w444:string)
                            }
                            frame "Command" {
                              n197 = property class="IMAQdx"(reference=w450, "ActiveAttribute"=w451) -> ()  [unwired: 1 in, 2 out]
                            }
                          }
                        }
                      }
                      n198 = Not(x=w394) -> (.not. x?=w392:bool)
                      n199 = Select(t=u32 9868950, s=w392, f=u32 0) -> (s? t:f=w391:u32)
                      n200 = property on="Tree" class="Tree (strict)"("Active Item Tag"=w395, "ActiveColNum"=1 ("Active Cell:Active Column Number"), "Cell String"=w396, "CellFontItalic"=w392, "CellFontBold"=w393, "CellFontColor"=w391) -> ()  [unwired: 2 in, 2 out]
                    }
                  }
                  frame #2 {
                    n201 = property class="IMAQdx"(reference=w453, "ActiveAttribute"=w452) -> ()  [unwired: 1 in, 2 out]
                    n202 = call <vilib>:"Unset Busy.vi"() -> ()  [unwired: 11 in, 1 out]
                  }
                }
              }
            }
          }
          event "Which cameras record": Value Change {
            n203 = event-data() -> ("NewVal"=w456:bool[])  [unwired: 1 in]
            n204 = Array Size(array=w458) -> (size(s)=w457:i32)
            n205 = Array Subset(array=w456, index=0, length=w457) -> (w454:bool[])
            n206 = property on="Which cameras record" class="Arr (strict)"("Value"=w454) -> ()  [unwired: 2 in, 2 out]
            n207 = property on="Which cameras record out" class="Arr (strict)"("Value"=w454) -> ()  [unwired: 2 in, 2 out]
          }
          event "Camera to address": Value Change {
            n208 = event-data() -> ("NewVal"=w461:i32)  [unwired: 1 in, 5 out]
            n209 = Decrement(x=w461) -> (x-1=w462:i32)
            n210 = property on="Camera to address out" class="DigNum (strict)"("Value"=w461) -> ()  [unwired: 2 in, 2 out]
            n211 = Index Array(array=w464, index=w462) -> (element=w463:T4)
            n212 = case shown="0" w461 {
              tunnel: w463 -> [_ w471]
              tunnel: w460 -> [_ w470]
              frame 0 {
                w468 = T7."Disabled and Grayed Out" ("Disabled")
                n213 = invoke on="Tree" class="Tree (strict)" method="Edit Tree Items.Delete"("Delete Children"=TRUE ("Delete Children?")) -> (error out=w466:errorcluster)  [unwired: 4 in, 4 out]
                n214 = call <vilib>:"Clear Errors.vi"("error in (no error)"=w466) -> ()  [unwired: 5 in, 2 out]
                n215 = property on="CameraU32" class="DigNum (strict)"("DisabledEnum"=w468) -> ()  [unwired: 2 in, 2 out]
                n216 = property on="CameraI64" class="DigNum (strict)"("DisabledEnum"=w468) -> ()  [unwired: 2 in, 2 out]
                n217 = property on="CameraDBL" class="DigNum (strict)"("DisabledEnum"=w468) -> ()  [unwired: 2 in, 2 out]
                n218 = property on="CameraString" class="Str"("DisabledEnum"=w468) -> ()  [unwired: 2 in, 2 out]
                n219 = property on="CameraEnum" class="Ring (strict)"("DisabledEnum"=w468) -> ()  [unwired: 2 in, 2 out]
                n220 = property on="CameraBool" class="Bool (strict)"("DisabledEnum"=w468) -> ()  [unwired: 2 in, 2 out]
                n221 = property on="CameraCommand" class="Str"("DisabledEnum"=w468) -> ()  [unwired: 2 in, 2 out]
                n222 = property on="Tree" class="Tree (strict)"("DisabledEnum"=w468) -> ()  [unwired: 2 in, 2 out]
              }
              frame 1, Default {
                n223 = stacked-sequence {
                  tunnel: w471 -> [_ w472 _]
                  frame #0 {
                    n224 = call <vilib>:"Set Busy.vi"() -> ()  [unwired: 10 in, 2 out]
                  }
                  frame #1 {
                    w481 = T7."Enabled" ("Disabled")
                    n225 = call <vilib>:"IMAQdx Enumerate Attributes.vi"("Visibility"=IMAQdx_Attribute_Visibility."Advanced", "Session In"=w472) -> ("error out"=w476:errorcluster, "Attribute Information Array"=w480:T9)  [unwired: 7 in, 1 out]
                    n226 = invoke on="Tree" class="Tree (strict)" method="Edit Tree Items.Delete"(error in=w476, "Delete Children"=TRUE ("Delete Children?")) -> (error out=w475:errorcluster)  [unwired: 3 in, 4 out]
                    n227 = call <vilib>:"Clear Errors.vi"("error in (no error)"=w475) -> ("error out"=w477:errorcluster)  [unwired: 5 in, 1 out]
                    n228 = for {
                      tunnel: w480 -> [w491] mode=indexing
                      tunnel: w477 -> [w484]
                      tunnel: [w483] -> w479
                      n229 = Unbundle(w491) -> ("Attribute Name"=w482:string)  [unwired: 3 out]
                      n230 = while {
                        shift-right: [w537] -> _
                        shift-left: w482 -> [w539]
                        tunnel: [w533] -> w488 mode=indexing
                        stop <- w534 stop-if-true
                        n231 = Match Pattern(string=w539, regular expression="::") -> (before substring=w533:string, after substring=w537:string, offset past match=w536:i32)  [unwired: 1 in, 1 out]
                        n232 = Equal?(x=w536, y=-1) -> (x = y?=w534:bool)
                      }
                      n233 = invoke on="Tree" class="Tree (strict)" method="Navigate Tree.Get Next"(error in=w484, "Tag"="") -> (error out=w483:errorcluster, "Navigate Tree:Get Next Item"=w486:string)  [unwired: 2 in, 2 out]
                      n234 = Array Size(array=w488) -> (size(s)=w489:i32)
                      n235 = Decrement(x=w489) -> (x-1=w485:i32)
                      n236 = for {
                        tunnel: w488 -> [w500] mode=indexing
                        shift-right: [w499] -> _
                        shift-left: "" -> [w498]
                        tunnel: w485 -> [w496]
                        shift-right: [w493] -> _
                        shift-left: w486 -> [w494]
                        tunnel: w482 -> [w492]
                        i -> [w495]
                        n237 = Greater Or Equal?(x=w495, y=w496) -> (x >= y?=w497:bool)
                        n238 = while {
                          shift-right: [w505] -> w493
                          shift-left: w494 -> [w506]
                          tunnel: w500 -> [w507]
                          tunnel: [w509] -> w499
                          tunnel: w498 -> [w508]
                          tunnel: w497 -> [w504]
                          tunnel: w492 -> [w502]
                          stop <- w511 stop-if-true
                          n239 = Equal?(x=w506, y=w507) -> (x = y?=w512:bool)
                          n240 = Equal?(x=w506, y="") -> (x = y?=w510:bool)
                          n241 = Select(t=w502, s=w504, f="") -> (s? t:f=w503:string)
                          n242 = Or(x=w512, y=w510) -> (x .or. y?=w511:bool)
                          n243 = case shown="True" w511 {
                            tunnel: w506 -> [w515 w523]
                            tunnel: w510 -> [_ w524]
                            tunnel: [w516 w522] -> w509
                            tunnel: w508 -> [w516 w521]
                            tunnel: w504 -> [_ w520]
                            tunnel: w507 -> [_ w519]
                            tunnel: [w514 w518] -> w505
                            tunnel: w503 -> [_ w517]
                            frame False {
                              n244 = invoke on="Tree" class="Tree (strict)" method="Navigate Tree.Get Next"("Tag"=w515) -> ("Navigate Tree:Get Next Item"=w514:string)  [unwired: 3 in, 3 out]
                            }
                            frame True {
                              n245 = case shown="True" w524 {
                                tunnel: w523 -> [w525 _]
                                tunnel: [w525 w528] -> w522
                                tunnel: w521 -> [_ w529]
                                tunnel: w520 -> [_ w531]
                                tunnel: w519 -> [_ w530]
                                tunnel: [w526 w528] -> w518
                                tunnel: w517 -> [_ w527]
                                frame False {
                                n246 = invoke on="Tree" class="Tree (strict)" method="Navigate Tree.Get Child"("Tag"=w525) -> ("Navigate Tree:Get Child"=w526:string)  [unwired: 3 in, 3 out]
                                }
                                frame True {
                                n247 = invoke on="Tree" class="Tree (strict)" method="Edit Tree Items.Add Item"("Parent Tag"=w529, "Child Position"=-1, "Left Cell"=w530, "Child Tag"=w527, "Child Only?"=w531) -> ("Edit Tree Items:Add Item"=w528:string)  [unwired: 4 in, 8 out]
                                }
                              }
                            }
                          }
                        }
                      }
                    }
                    n248 = invoke on="Tree" class="Tree (strict)" method="Open/Close.Open/Close All"(error in=w479, "Open"=FALSE ("Open?")) -> ()  [unwired: 2 in, 4 out]
                    n249 = property on="CameraU32" class="DigNum (strict)"("DisabledEnum"=w481) -> ()  [unwired: 2 in, 2 out]
                    n250 = property on="CameraI64" class="DigNum (strict)"("DisabledEnum"=w481) -> ()  [unwired: 2 in, 2 out]
                    n251 = property on="CameraDBL" class="DigNum (strict)"("DisabledEnum"=w481) -> ()  [unwired: 2 in, 2 out]
                    n252 = property on="CameraString" class="Str"("DisabledEnum"=w481) -> ()  [unwired: 2 in, 2 out]
                    n253 = property on="CameraEnum" class="Ring (strict)"("DisabledEnum"=w481) -> ()  [unwired: 2 in, 2 out]
                    n254 = property on="CameraBool" class="Bool (strict)"("DisabledEnum"=w481) -> ()  [unwired: 2 in, 2 out]
                    n255 = property on="CameraCommand" class="Str"("DisabledEnum"=w481) -> ()  [unwired: 2 in, 2 out]
                    n256 = property on="Tree" class="Tree (strict)"("DisabledEnum"=w481) -> ()  [unwired: 2 in, 2 out]
                  }
                  frame #2 {
                    n257 = call <vilib>:"Unset Busy.vi"() -> ()  [unwired: 11 in, 1 out]
                  }
                }
                n258 = Generate User Event(user event=w470, event data cluster=TRUE ("event data")) -> ()  [unwired: 2 in, 2 out]
              }
            }
          }
          event "Offset and gain": Value Change {
            n259 = event-data() -> ("NewVal"=w541:dbl[][])  [unwired: 1 in, 5 out]
            n260 = property on="Offset gain out" class="Arr (strict)"("Value"=w541) -> ()  [unwired: 2 in, 2 out]
          }
          event "RGB Channels in": Value Change {
            n261 = event-data() -> ("NewVal"=w543:T2)  [unwired: 1 in, 5 out]
            n262 = property on="RGB Channels out" class="Arr (strict)"("Value"=w543) -> ()  [unwired: 2 in, 2 out]
          }
          event "Camera orientation": Value Change {
            n263 = event-data() -> ("NewVal"=w545:T3)  [unwired: 1 in, 5 out]
            n264 = property on="Camera orientation out" class="Arr (strict)"("Value"=w545) -> ()  [unwired: 2 in, 2 out]
          }
          event "Autorange Red", "Autorange Green", "Autorange Blue": Value Change {
            n265 = event-data() -> ("CtlRef"=w548:refnum<vi>, "CtlRef"=w556:refnum<vi>, "NewVal"=w557:bool)  [unwired: 1 in, 3 out]
            n266 = property on="RGB Channels in" class="Arr (strict)"() -> ("Value"=w555:T2)  [unwired: 2 in, 2 out]
            n267 = control-ref of="Autorange Blue"() -> (w549:refnum<vi>)
            n268 = control-ref of="Autorange Red"() -> (w551:refnum<vi>)
            n269 = control-ref of="Autorange Green"() -> (w550:refnum<vi>)
            n270 = case shown="True" w557 {
              tunnel: w556 -> [_ w595]
              frame False {
              }
              frame True {
                n271 = property class="Bool (strict)"(reference=w595, "Value"=FALSE) -> ()  [unwired: 1 in, 2 out]
              }
            }
            n272 = Build Array(w551, w550, w549) -> (w547:refnum<vi>[])
            n273 = for {
              tunnel: w548 -> [w560]
              tunnel: w547 -> [w561] mode=indexing
              tunnel: [w558] -> w546
              i -> [w558]
              stop <- w559 stop-if-true
              n274 = Equal?(x=w561, y=w560) -> (x = y?=w559:bool)
            }
            n275 = Index Array(array=w555, index=w546) -> (element=w554:T10)
            n276 = case shown="\"Camera 1\", Default" w554 {
              selector: w554 -> [_ w586]
              tunnel: w553 -> [_ w593]
              tunnel: w546 -> [_ w562]
              frame "None" {
              }
              frame "Camera 1", Default {
                n277 = Decrement(x=w586) -> (x-1=w585:T10)
                n278 = Index Array(array=w593, index=w585) -> (element=w584:T1)
                n279 = call "IMAQ ImageToArray"("Image"=w584) -> ("Image Pixels (I16)"=w583:i16[][])  [unwired: 3 in, 4 out]
                n280 = Array Size(array=w583) -> (size(s)=w582:i32[])
                n281 = Multiply Array Elements(1:w582) -> (0:w571:i32)
                n282 = To Double Precision Float(number=w571) -> (double precision float=w572:dbl)
                n283 = To Double Precision Float(number=w571) -> (double precision float=w574:dbl)
                n284 = Reshape Array(w583, w571) -> (w581:i16[])
                n285 = Sort 1D Array(array=w581) -> (sorted array=w580:i16[])
                n286 = Multiply(x=w572, y=0.99) -> (x*y=w578:dbl)
                n287 = Multiply(x=w574, y=0.01) -> (x*y=w575:dbl)
                n288 = Round To Nearest(number=w578) -> (nearest integer value=w577:dbl)
                n289 = Round To Nearest(number=w575) -> (nearest integer value=w570:dbl)
                n290 = To Long Integer(number=w570) -> (32bit integer=w569:i32)
                n291 = To Long Integer(number=w577) -> (32bit integer=w576:i32)
                n292 = Index Array(array=w580, index #1=w576, index #2=w569) -> (element #1=w567:i16, element #2=w566:i16)
                n293 = To Double Precision Float(number=w567) -> (double precision float=w565:dbl)
                n294 = To Double Precision Float(number=w566) -> (double precision float=w564:dbl)
                n295 = Subtract(x=w565, y=w564) -> (x-y=w592:dbl)
                n296 = Negate(x=w564) -> (-x=w587:dbl)
                n297 = Reciprocal(x=w592) -> (1/x=w563:dbl)
                n298 = property on="Offset and gain" class="Arr (strict)"() -> ("Value"=w590:dbl[][])  [unwired: 2 in, 2 out]
                n299 = Multiply(x=255.0, y=w563) -> (x*y=w588:dbl)
                n300 = Build Array(w587, w588) -> (w568:dbl[])
                n301 = Replace Array Subset(array=w590, new element=w568, index (row)=w562) -> (w589:dbl[][])  [unwired: 1 in]
                n302 = property on="Offset and gain" class="Arr (strict)"("Val(Sgnl)"=w589) -> ()  [unwired: 2 in, 2 out]
              }
            }
          }
          event "CameraU32", "CameraI64", "CameraDBL", "CameraString", "CameraBool", "CameraEnum", "CameraCommand": Value Change {
            n303 = event-data() -> ("CtlRef"=w599:refnum<vi>, "NewVal"=w601:variant)  [unwired: 1 in]
            n304 = flat-sequence {
              tunnel: w601 -> [w608]
              tunnel: w600 -> [w607]
              tunnel: w599 -> [w606]
              tunnel: w598 -> [w605]
              tunnel: w596 -> [w643]
              frame #0 {
                n305 = property on="Camera to address" class="DigNum (strict)"() -> ("Value"=w603:i32)  [unwired: 2 in, 2 out]
                n306 = Decrement(x=w603) -> (x-1=w602:i32)
                n307 = Index Array(array=w605, index=w602) -> (element=w604:T4)
                n308 = for {
                  tunnel: w607 -> [w613] mode=indexing
                  tunnel: w606 -> [w612]
                  tunnel: [w610] -> w609
                  i -> [w610]
                  stop <- w611 stop-if-true
                  n309 = Equal?(x=w612, y=w613) -> (x = y?=w611:bool)
                }
                n310 = case shown="4" w609 {
                  tunnel: w608 -> [w617 w621 w625 w629 w633 w637 w641]
                  tunnel: w604 -> [w616 w620 w624 w628 w632 w636 w640]
                  frame 0, Default {
                    n311 = Variant To Data(type=u32 0, Variant=w617) -> (data=w615:u32)  [unwired: 1 in, 1 out]
                    n312 = property class="IMAQdx"(reference=w616, "ValueU32"=w615) -> ()  [unwired: 1 in, 2 out]
                  }
                  frame 1 {
                    n313 = Variant To Data(type=i64 0, Variant=w621) -> (data=w619:i64)  [unwired: 1 in, 1 out]
                    n314 = property class="IMAQdx"(reference=w620, "ValueI64"=w619) -> ()  [unwired: 1 in, 2 out]
                  }
                  frame 2 {
                    n315 = Variant To Data(type=0.0, Variant=w625) -> (data=w623:dbl)  [unwired: 1 in, 1 out]
                    n316 = property class="IMAQdx"(reference=w624, "ValueDBL"=w623) -> ()  [unwired: 1 in, 2 out]
                  }
                  frame 3 {
                    n317 = Variant To Data(type="", Variant=w629) -> (data=w627:string)  [unwired: 1 in, 1 out]
                    n318 = property class="IMAQdx"(reference=w628, "ValueString"=w627) -> ()  [unwired: 1 in, 2 out]
                  }
                  frame 4 {
                    n319 = Variant To Data(type=u32 0, Variant=w633) -> (data=w631:u32)  [unwired: 1 in, 1 out]
                    n320 = property class="IMAQdx"(reference=w632, "ValueU32"=w631) -> ()  [unwired: 1 in, 2 out]
                  }
                  frame 5 {
                    n321 = Variant To Data(type=TRUE, Variant=w637) -> (data=w635:bool)  [unwired: 1 in, 1 out]
                    n322 = property class="IMAQdx"(reference=w636, "ValueBool"=w635) -> ()  [unwired: 1 in, 2 out]
                  }
                  frame 6 {
                    n323 = Variant To Data(type="", Variant=w641) -> (data=w639:string)  [unwired: 1 in, 1 out]
                    n324 = property class="IMAQdx"(reference=w640, "ValueString"=w639) -> ()  [unwired: 1 in, 2 out]
                  }
                }
              }
              frame #1 {
                n325 = Generate User Event(user event=w643, event data cluster=TRUE ("event data")) -> ()  [unwired: 2 in, 2 out]
              }
            }
          }
          event "Refresh": Value Change {
            n326 = event-data() -> ("NewVal"=w646:bool)  [unwired: 1 in, 5 out]
            n327 = case shown="True" w646 {
              tunnel: w645 -> [_ w648]
              frame False {
              }
              frame True {
                n328 = Generate User Event(user event=w648, event data cluster=TRUE ("event data")) -> ()  [unwired: 2 in, 2 out]
                n329 = property on="Refresh" class="Bool (strict)"("Value"=FALSE ("Trigger")) -> ()  [unwired: 2 in, 2 out]
              }
            }
          }
        }
      }
    }
    frame #2 {
      n330 = Destroy User Event(user event=w650) -> ()  [unwired: 1 in, 1 out]
    }
  }
